vi "Register for Events (Multiple PyObjects).vi"(8 "error in (no error)":errorcluster, 9 "PyObjects":T1[](array[typedef]), 11 "JKI_Python_Server in":refnum<class "Server.lvclass">) -> (0 "error out":errorcluster, 1 "Python":T3, 3 "JKI_Python_Server out":refnum<class "Server.lvclass">)   [LabVIEW 2013, in "JKI_Python_Bridge_for_LV.lvlib" / "Server.lvclass"]
uses:
  Server.lvclass
  Type Definitions/Python Method Call - Event Registration.ctl
  Call/Call.lvclass
  Type Definitions/Public Events - Cluster.ctl
  Type Definitions/Python Object and Method Names - Cluster.ctl
  Type Definitions/Python Method.ctl
  PyObject/PyObject.lvclass
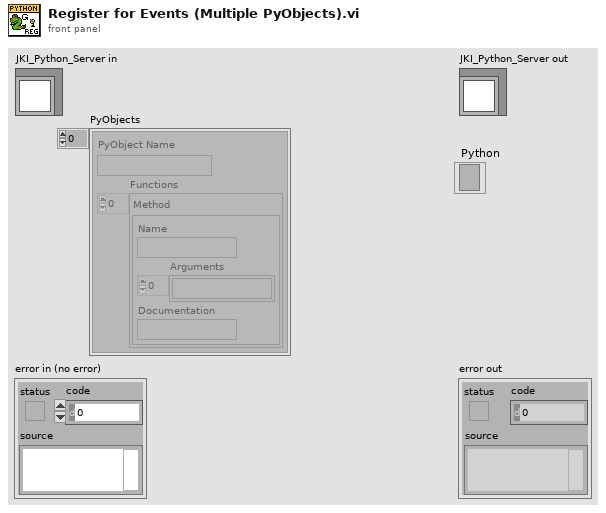
[diagram p1: front panel]
types:
  T1 = typedef "JKI_Python_Bridge_for_LV.lvlib/Server.lvclass/Python Object and Method Names - Cluster.ctl" = cluster{"PyObject Name":string, "Functions":T2[]}
  T2 = typedef "JKI_Python_Bridge_for_LV.lvlib/Server.lvclass/Python Method.ctl" = cluster{"Name":string, "Arguments":string[], "Documentation":string}
  T3 = typedef "JKI_Python_Bridge_for_LV.lvlib/Server.lvclass/Python Method Call - Event Registration.ctl" = refnum<event-registration>
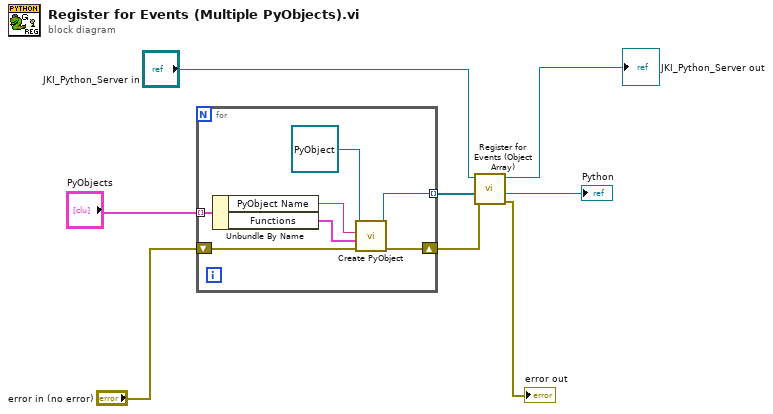
[diagram p0: block diagram]
diagram:
  n1 = for {
    tunnel: [w14] -> w1 mode=indexing
    shift-right: [w12] -> w3
    shift-left: "error in (no error)" -> [w13]
    tunnel: "PyObjects" -> [w11] mode=indexing
    n2 = Unbundle By Name(w11) -> ("PyObject Name"=w10:string, "Functions"=w9:T2[])
    n3 = call "Create PyObject.vi"("error in (no error)"=w13, "Methods"=w9, "PyObject Name"=w10, "Node in"=refnum<class "PyObject.lvclass"> refnum) -> ("error out"=w12:errorcluster, "Node out"=w14:refnum<class "PyObject.lvclass">)  [unwired: 6 in]
  }
  n4 = call "Register for Events (Object Array).vi"("error in (no error)"=w3, "PyObject []"=w1, "JKI_Python_Server in"="JKI_Python_Server in") -> ("error out"=→"error out":errorcluster, "Python Event"=→"Python":T3, "JKI_Python_Server out"=→"JKI_Python_Server out":refnum<class "Server.lvclass">)  [unwired: 6 in]
